vi "Initialize.vi"(0 "Room Service Monitor Model in":refnum<class "Room Service Monitor Model.lvclass">, 11 "error in (no error)":errorcluster) -> (4 "Room Service Monitor Model out":refnum<class "Room Service Monitor Model.lvclass">, 15 "error out":errorcluster)   [LabVIEW 2023, in "Room Service Monitor Model.lvlib" / "Room Service Monitor Model.lvclass"]
uses:
  Room Service Monitor Model.lvclass
  Room Service Monitor Model.lvclass/Room Service Monitor Model.ctl
  <vilib>/ActorFramework/Actor/Actor.lvclass
  Room Service Monitor UI/Room Service Monitor UI/Room Service Monitor UI.lvclass
  C:/Users/bhaghyaraj/Trainings/NI Actor Framework/SDLC/UI Base/UI Base/UI Base.lvclass
  C:/Program Files/National Instruments/LabVIEW 2023/vi.lib/ActorFramework/Actor/Actor.lvclass
  C:/Users/bhaghyaraj/Trainings/NI Actor Framework/SDLC/Room Service Monitor UI/Room Service Monitor UI/Room Service Monitor UI.lvclass
  C:/Users/bhaghyaraj/Trainings/NI Actor Framework/SDLC/Model Base/Model Base/Model Base.lvclass
  C:/Users/bhaghyaraj/Trainings/NI Actor Framework/SDLC/Interfaces/Model Base/Incoming Model Base Interface.lvclass
  C:/Users/bhaghyaraj/Trainings/NI Actor Framework/SDLC/Room Service Monitor Model/Room Service Monitor Model/Room Service Monitor Model.lvclass
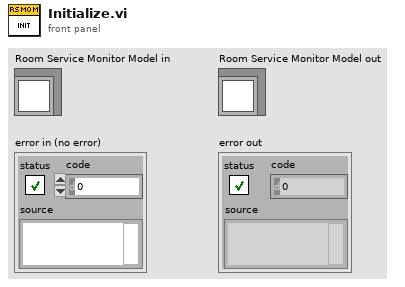
[diagram p1: front panel]
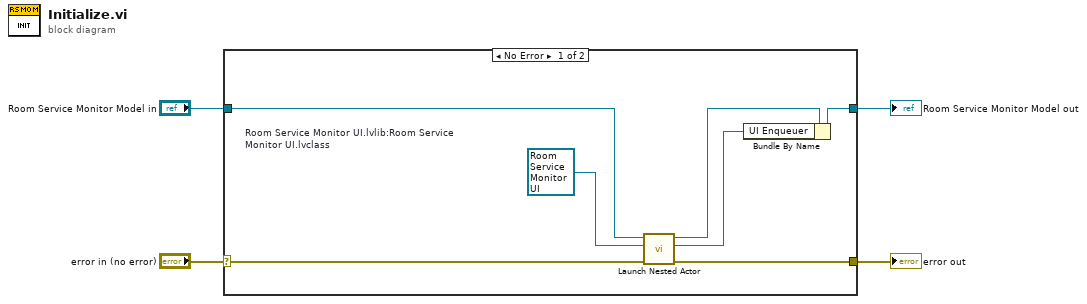
[diagram p0: block diagram]
diagram:
  n1 = case shown="No Error" "error in (no error)" {
    selector: "error in (no error)" -> [w6 w13]
    tunnel: [w11 w13] -> w2
    tunnel: [w8 w12] -> w1
    tunnel: "Room Service Monitor Model in" -> [w10 w12]
    frame No Error {
      w5 = refnum<class "Room Service Monitor UI.lvclass"> refnum  # Room Service Monitor UI.lvlib:Room Service Monitor UI.lvclass
      n2 = call <vilib>:"Launch Nested Actor.vi"("error in (no error)"=w6, "Nested Actor"=w5, "Caller Actor in"=w10) -> ("error out"=w11:errorcluster, "Nested Actor's Enqueuer"=w7:refnum<class "Message Enqueuer.lvclass">, "Caller Actor out"=w9:refnum<class "Room Service Monitor Model.lvclass">)  [unwired: 6 in]
      n3 = Bundle By Name(cluster=w9, "UI Enqueuer"=w7) -> (w8:refnum<class "Room Service Monitor Model.lvclass">)
    }
    frame Error {
    }
  }
  "error out" <- w2
  "Room Service Monitor Model out" <- w1
